vi "Wait.vi"(8 "Error In":errorcluster, 9 "WaitOnError":bool, 11 "milliseconds to wait":u32) -> (0 "Error Out":errorcluster)   [LabVIEW 2019, in "Utilities.lvlib"]
uses:
  Utilities.lvlib
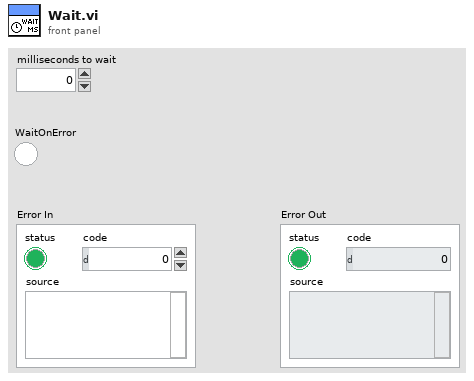
[diagram p1: front panel]
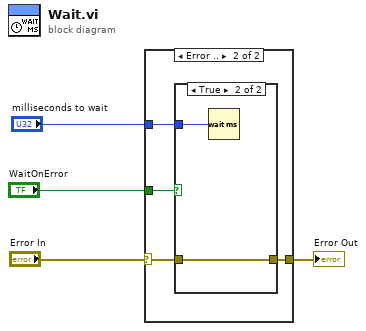
[diagram p0: block diagram]
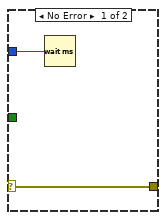
[diagram p2: hidden frame]
diagram:
  n1 = case shown="Error .." "Error In" {
    selector: "Error In" -> [w5 w10]
    tunnel: "milliseconds to wait" -> [w6 w8]
    tunnel: [w5 w7] -> w2
    tunnel: "WaitOnError" -> [_ w9]
    frame No Error {
      n2 = Wait (ms)(milliseconds to wait=w6) -> ()  [unwired: 1 out]
    }
    frame Error {
      n3 = case shown="True" w9 {
        tunnel: w10 -> [w11 w12]
        tunnel: w8 -> [_ w13]
        tunnel: [w11 w12] -> w7
        frame False {
        }
        frame True {
          n4 = Wait (ms)(milliseconds to wait=w13) -> ()  [unwired: 1 out]
        }
      }
    }
  }
  "Error Out" <- w2
